vi "PXI-Find Min AO Delay.vi"(0 "Fs (Hz)":dbl, 5 "AO Channels":i32[](array[numeric])) -> (4 "Samples":i32)   [LabVIEW 2020]
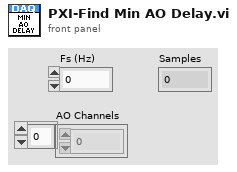
[diagram p1: front panel]
types:
  T1 = cluster{"DAQChan to PhysDev":i32[][], "PhysDev to DAQChan":i32[][]}
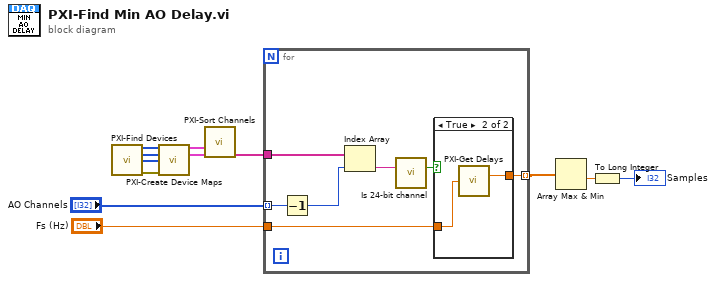
[diagram p0: block diagram]
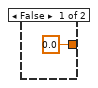
[diagram p2: hidden frame]
diagram:
  n1 = call "PXI-Find Devices.vi"() -> ("Num AO"=w10:i32[], "Num AI"=w9:i32[], "Slot Num"=w12:u32[], "error out"=w11:errorcluster)  [unwired: 12 in]
  n2 = call "PXI-Create Device Maps.vi"("Num AO"=w10, "Num AI"=w9, "Slot Num"=w12, "error in (no error)"=w11) -> ("AO Map"=w8:T1, "AI Map"=w7:T1)  [unwired: 9 in, 1 out]
  n3 = call "PXI-Sort Channels.vi"("AO Map"=w8, "AI Map"=w7) -> ("Sorted physical channels"=w5:tag[])  [unwired: 12 in, 1 out]
  n4 = for {
    tunnel: "AO Channels" -> [w19] mode=indexing
    tunnel: w5 -> [w18]
    tunnel: [w16] -> w4 mode=indexing
    tunnel: "Fs (Hz)" -> [w15]
    n5 = Decrement(x=w19) -> (x-1=w17:i32)
    n6 = Index Array(array=w18, index=w17) -> (element=w14:tag)
    n7 = call "Is 24-bit channel.vi"("DAQmx Physical Channel"=w14) -> ("is 24bit?"=w13:bool)  [unwired: 12 in, 2 out]
    n8 = case shown="True" w13 {
      tunnel: [0.0 ("AO delay (samples)") w22] -> w16
      tunnel: w15 -> [_ w21]
      frame False {
      }
      frame True {
        n9 = call "PXI-Get Delays.vi"("AO Rate (Samples/s)"=w21) -> ("AO delay (samples)"=w22:dbl)  [unwired: 13 in, 1 out]
      }
    }
  }
  n10 = Array Max & Min(array=w4) -> (min value=w3:dbl)  [unwired: 3 out]
  n11 = To Long Integer(number=w3) -> (32bit integer=→"Samples":i32)
